vi "gxml_BlindExtractType.vi"(6 "Encaps Array Info":T1, 8 "error in":errorcluster, 11 "XML Line":string) -> (0 "error out":errorcluster, 1 "Item Name":cluster{"Hierarchy":string, "Item Name":string}, 2 "Extracted Content":string, 3 "Extracted Type":string, 4 "Encaps Array Info Out":T1)   [LabVIEW 2011, in "Third Party VIs.lvlib" / "GXML.lvlib"]
uses:
  <vilib>/regexp/Match Regular Expression.xnode
  GXML.lvlib
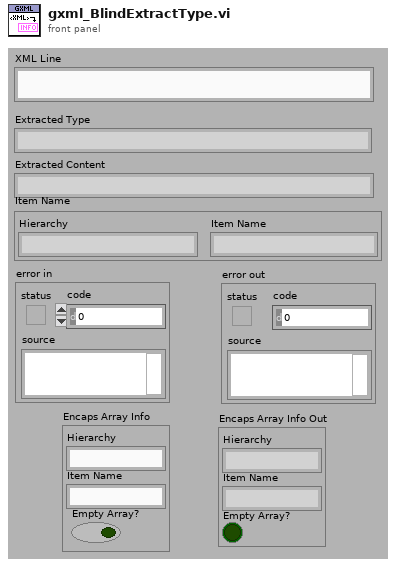
[diagram p1: front panel]
types:
  T1 = cluster{"Hierarchy":string, "Item Name":string, "Empty Array?":bool}
  T2 = cluster{"token string":string, "token string":string}
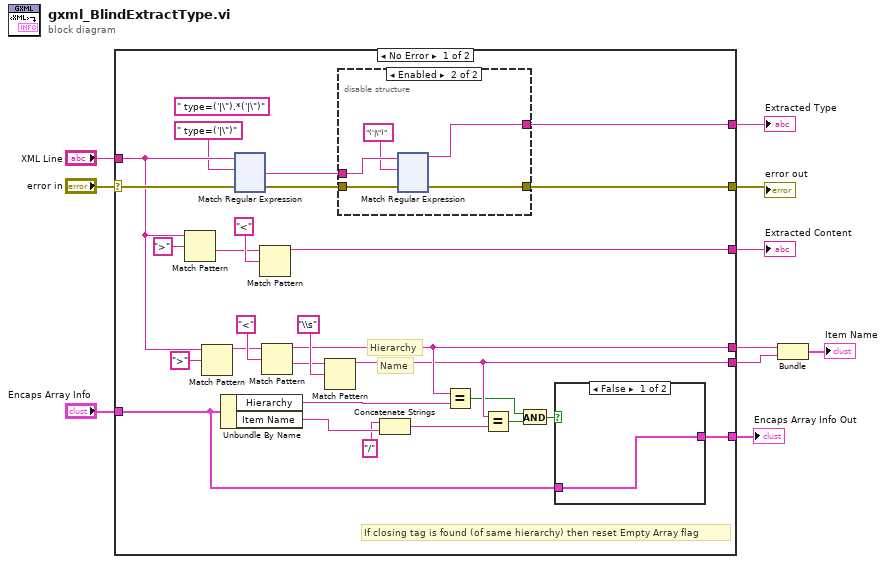
[diagram p0: block diagram]
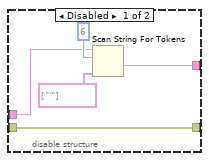
[diagram p2: hidden frame]
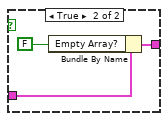
[diagram p3: hidden frame]
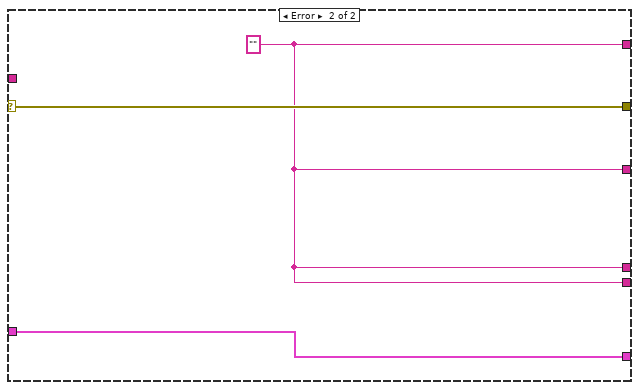
[diagram p4: hidden frame]
diagram:
  n1 = case shown="No Error" "error in" {
    selector: "error in" -> [w36 w276]
    tunnel: [w37 w275] -> w10
    tunnel: "XML Line" -> [w18 _]
    tunnel: [w13 w276] -> w8
    tunnel: [w15 w275] -> w6
    tunnel: [w30 w275] -> w5
    tunnel: [w25 w275] -> w4
    tunnel: "Encaps Array Info" -> [w21 w274]
    tunnel: [w20 w274] -> w1
    frame No Error {
      (unwired) " type=('|\").*('|\")"
      # "If closing tag is found (of same hierarchy) then reset Empty Array flag"
      # "Name"
      # "Hierarchy"
      n2 = Match Pattern(string=w18, regular expression=">") -> (after substring=w16:string)  [unwired: 1 in, 3 out]
      n3 = Match Pattern(string=w18, regular expression=">") -> (before substring=w32:string)  [unwired: 1 in, 3 out]
      n4 = Unbundle By Name(w21) -> ("Hierarchy"=w29:string, "Item Name"=w28:string)
      n5 = xnode "Match Regular Expression"("input string"=w18, "regular expression"=" type=('|\")", "error in"=w36) -> ("after match"=w11:string, "error out"=w14:errorcluster)  [unwired: 3 in, 3 out]
      n6 = Match Pattern(string=w16, regular expression="<") -> (before substring=w15:string)  [unwired: 1 in, 3 out]
      n7 = Match Pattern(string=w32, regular expression="<") -> (before substring=w30:string, after substring=w34:string)  [unwired: 1 in, 2 out]
      n8 = Match Pattern(string=w34, regular expression="\\s") -> (before substring=w25:string)  [unwired: 1 in, 3 out]
      n9 = disable-structure shown="Enabled" {
        disable-tunnel: [w40 w43] -> w37
        disable-tunnel: w11 -> [w39 w45]
        disable-tunnel: [w38 w46] -> w13
        disable-tunnel: w14 -> [w38 w47]
        frame Disabled {
          n10 = Scan String For Tokens(6:string[] ["'"] ("delimiters (\\s,\\t,\\r,\\n)"), 8:6 ("offset"), 9:w39) -> (1:w40:string)  [unwired: 3 in, 3 out]
        }
        frame Enabled {
          n11 = xnode "Match Regular Expression"("input string"=w45, "regular expression"="('|\")", "error in"=w47) -> ("before match"=w43:string, "error out"=w46:errorcluster)  [unwired: 3 in, 3 out]
        }
      }
      n12 = Concatenate Strings("/" ("string"), w28) -> (w26:string)
      n13 = Equal?(x=w30, y=w29) -> (x = y?=w23:bool)
      n14 = Equal?(x=w25, y=w26) -> (x = y?=w24:bool)
      n15 = And(x=w23, y=w24) -> (x .and. y?=w22:bool)
      n16 = case shown="False" w22 {
        tunnel: w21 -> [w159 w162]
        tunnel: [w159 w160] -> w20
        frame False {
        }
        frame True {
          n17 = Bundle By Name(cluster=w162, "Empty Array?"=FALSE) -> (w160:T1)
        }
      }
    }
    frame Error {
      w275 = "" ("token string")
    }
  }
  "Extracted Type" <- w10
  "error out" <- w8
  "Extracted Content" <- w6
  "Encaps Array Info Out" <- w1
  n18 = Bundle("token string"=w5, "token string"=w4) -> (→"Item Name":T2)  [unwired: 1 in]
